vi "Decimate Map.vi"(11 "Map":T2={"Width"=250, "Height"=250, "Iterations"=256, "Top Left Coordinate"=-2.5+1.0i, "Bottom Right Coordinate"=1.0-1.0i}) -> (3 "Decimated Map":T1(array[cluster]))   [LabVIEW 2016, in "Map.lvclass"]
uses:
  Map.lvclass
panel:
  out "Numeric":i32
  out "Imaginary Part Distance 2":dbl
  out "Real Part Distance":dbl
  out "Re 1":dbl
  out "Im 1":dbl
  out "Re 2":dbl
  out "Im 2":dbl
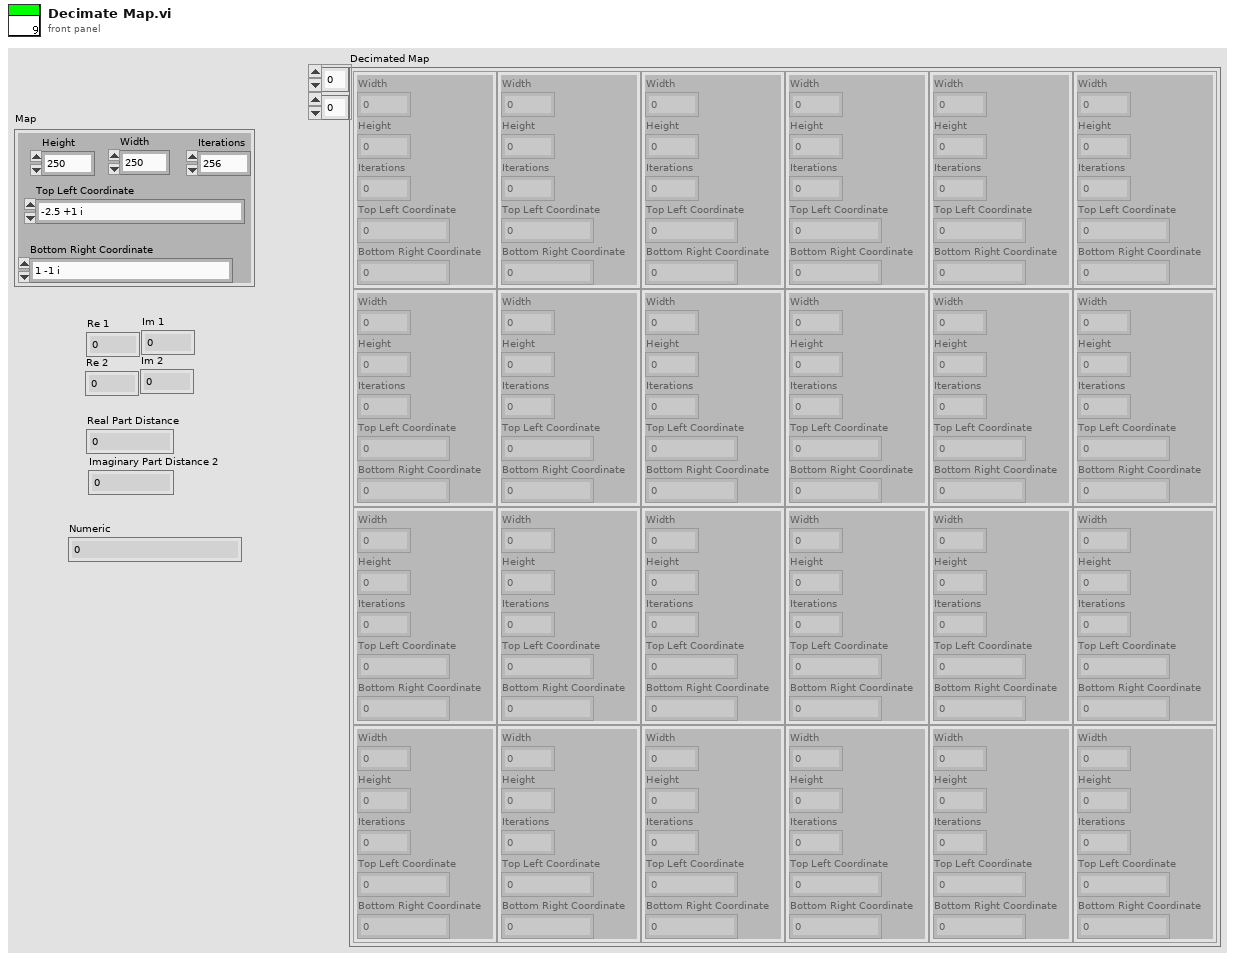
[diagram p1: front panel]
types:
  T1 = cluster{"Width":i32, "Height":i32, "Iterations":u16, "Top Left Coordinate":cdb, "Bottom Right Coordinate":cdb}[][]
  T2 = cluster{"Width":i32, "Height":i32, "Iterations":u16, "Top Left Coordinate":cdb, "Bottom Right Coordinate":cdb}
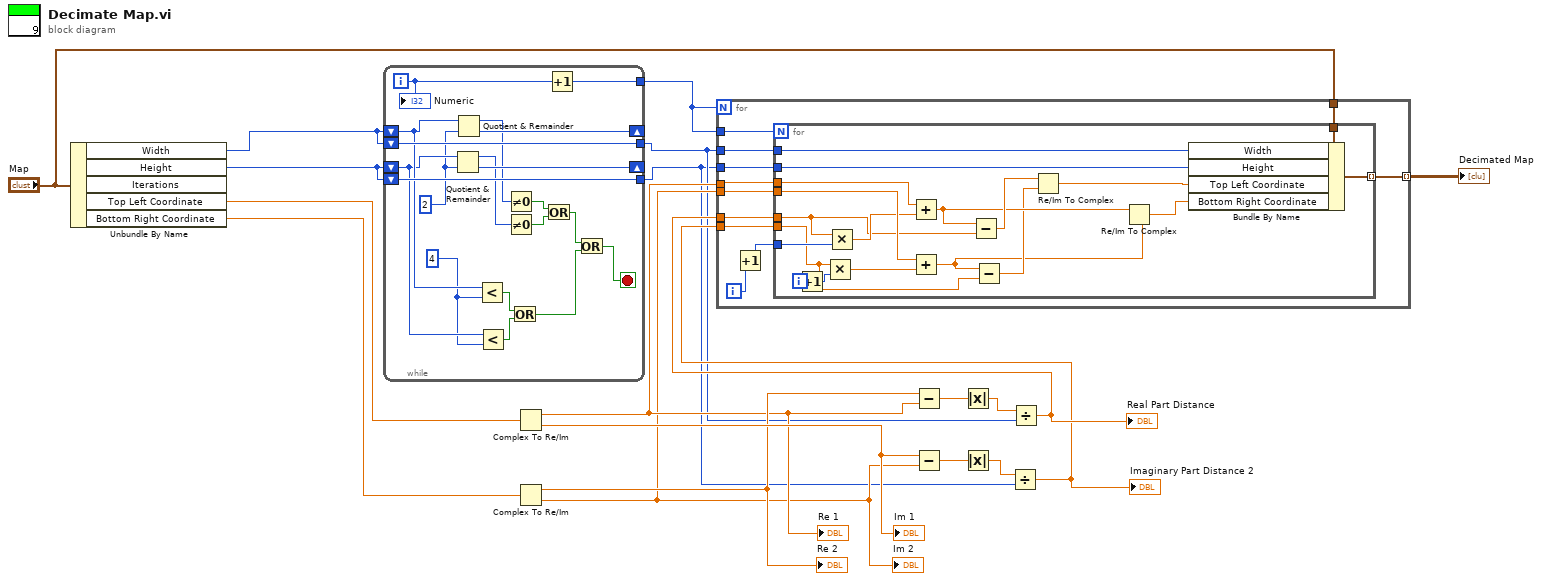
[diagram p0: block diagram]
diagram:
  n1 = Unbundle By Name("Map") -> ("Width"=w19:i32, "Height"=w18:i32, "Top Left Coordinate"=w16:cdb, "Bottom Right Coordinate"=w15:cdb)  [unwired: 1 out]
  n2 = while {
    shift-right: [w34] -> _
    shift-left: w19 -> [w28]
    shift-right: [w33] -> _
    shift-left: w18 -> [w27]
    shift-left: w19 -> [w38]
    shift-left: w18 -> [w37]
    tunnel: [w38] -> w3
    tunnel: [w37] -> w2
    tunnel: [w35] -> w4
    i -> [w36]
    stop <- w20 stop-if-true
    w23 = 4 ("y")
    w26 = 2 ("y")
    n3 = Quotient & Remainder(x=w27, y=w26) -> (x-y*floor(x/y)=w31:i32, floor(x/y)=w33:i32)
    n4 = Quotient & Remainder(x=w28, y=w26) -> (x-y*floor(x/y)=w32:i32, floor(x/y)=w34:i32)
    n5 = Less?(x=w28, y=w23) -> (x < y?=w25:bool)
    n6 = Less?(x=w27, y=w23) -> (x < y?=w24:bool)
    n7 = Not Equal To 0?(x=w32) -> (x != 0?=w30:bool)
    n8 = Not Equal To 0?(x=w31) -> (x != 0?=w29:bool)
    n9 = Or(x=w25, y=w24) -> (x .or. y?=w21:bool)
    n10 = Or(x=w30, y=w29) -> (x .or. y?=w22:bool)
    n11 = Increment(x=w36) -> (x+1=w35:i32)
    n12 = Or(x=w22, y=w21) -> (x .or. y?=w20:bool)
    "Numeric" <- w36
  }
  n13 = Complex To Re/Im(x + iy=w16) -> (x=w8:dbl, y=w10:dbl)
  "Re 1" <- w8
  "Im 1" <- w10
  n14 = Complex To Re/Im(x + iy=w15) -> (x=w9:dbl, y=w6:dbl)
  "Re 2" <- w9
  "Im 2" <- w6
  n15 = Subtract(x=w9, y=w8) -> (x-y=w11:dbl)
  n16 = Subtract(x=w10, y=w6) -> (x-y=w14:dbl)
  n17 = Absolute Value(x=w11) -> (abs(x)=w12:dbl)
  n18 = Absolute Value(x=w14) -> (abs(x)=w13:dbl)
  n19 = Divide(x=w13, y=w2) -> (x/y=w5:dbl)
  "Imaginary Part Distance 2" <- w5
  n20 = Divide(x=w12, y=w3) -> (x/y=w7:dbl)
  "Real Part Distance" <- w7
  n21 = for {
    N: w4 -> [_]
    tunnel: w2 -> [w49]
    tunnel: w3 -> [w48]
    tunnel: "Map" -> [w47]
    tunnel: [w46] -> w1 mode=indexing
    tunnel: w4 -> [w45]
    tunnel: w8 -> [w44]
    tunnel: w7 -> [w43]
    tunnel: w5 -> [w42]
    tunnel: w6 -> [w41]
    i -> [w40]
    n22 = Increment(x=w40) -> (x+1=w39:i32)
    n23 = for {
      N: w45 -> [_]
      tunnel: w49 -> [w68]
      tunnel: w48 -> [w67]
      tunnel: w47 -> [w66]
      tunnel: [w61] -> w46 mode=indexing
      tunnel: w44 -> [w62]
      tunnel: w43 -> [w52]
      tunnel: w42 -> [w51]
      tunnel: w41 -> [w63]
      tunnel: w39 -> [w64]
      i -> [w65]
      n24 = Increment(x=w65) -> (x+1=w50:i32)
      n25 = Multiply(x=w51, y=w50) -> (x*y=w54:dbl)
      n26 = Multiply(x=w52, y=w64) -> (x*y=w53:dbl)
      n27 = Add(x=w62, y=w53) -> (x+y=w57:dbl)
      n28 = Add(x=w63, y=w54) -> (x+y=w55:dbl)
      n29 = Subtract(x=w57, y=w52) -> (x-y=w58:dbl)
      n30 = Subtract(x=w55, y=w51) -> (x-y=w56:dbl)
      n31 = Re/Im To Complex(1:w56, 2:w58) -> (0:w60:cdb)
      n32 = Re/Im To Complex(1:w55, 2:w57) -> (0:w59:cdb)
      n33 = Bundle By Name(cluster=w66, "Width"=w67, "Height"=w68, "Top Left Coordinate"=w60, "Bottom Right Coordinate"=w59) -> (w61:T2)
    }
  }
  "Decimated Map" <- w1
